vi "Sub - Create Vector.vi"(0 "Vector Start (0 +0i)":cdb, 5 "Vector End":cdb) -> (4 "Vector Points":cdb[](array[numeric]))   [LabVIEW 2015]
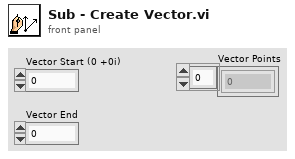
[diagram p1: front panel]
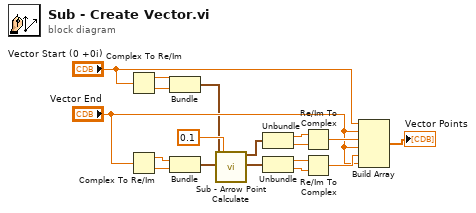
[diagram p0: block diagram]
diagram:
  n1 = Complex To Re/Im(x + iy="Vector Start (0 +0i)") -> (x=w2:dbl, y=w4:dbl)
  n2 = Complex To Re/Im(x + iy="Vector End") -> (x=w7:dbl, y=w8:dbl)
  n3 = Bundle(w2, w4) -> (w1:cluster{dbl, dbl})  [unwired: 1 in]
  n4 = Bundle(w7, w8) -> (w9:cluster{dbl, dbl})  [unwired: 1 in]
  n5 = call "Sub - Arrow Point Calculate.vi"("original position"=w1, "new position"=w9, "tail length(10)"=0.1) -> ("Tail endpoint 1"=w10:cluster{dbl, dbl}, "Tail endpoint 2"=w11:cluster{dbl, dbl})  [unwired: 15 in]
  n6 = Unbundle(w10) -> (w13:dbl, w12:dbl)
  n7 = Unbundle(w11) -> (w14:dbl, w15:dbl)
  n8 = Re/Im To Complex(1:w12, 2:w13) -> (0:w17:cdb)
  n9 = Re/Im To Complex(1:w15, 2:w14) -> (0:w16:cdb)
  n10 = Build Array("Vector Start (0 +0i)", "Vector End", w17, "Vector End", w16, "Vector End") -> (→"Vector Points":cdb[])
